vi "Ball Intake Logging Values.vi"() -> ()   [LabVIEW 2016]
panel:
  out "Commanded Intake Motor Value":dbl
  in  "Manual Reverse Intake":bool
  in  "Toggle Ball Intake":bool
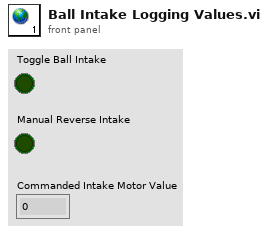
[diagram p1: front panel]
diagram:
